vi "Set Endpoints.vi"(8 "Color":u32(colorbox), 9 "B":refnum<class "Point.lvclass">, 10 "A":refnum<class "Point.lvclass">, 11 "Line in":refnum<class "Line example.lvclass">) -> (3 "Line out":refnum<class "Line example.lvclass">)   [LabVIEW 2018, in "Line example.lvclass"]
doc: "Set the endpoints and color of the line."
uses:
  Line example.lvclass
  e:/builds/penguin/labview/branches/2018/dev/dist64/examples/Object-Oriented Programming/Graphics/Graphic/Graphic.lvclass
  Point/Point.lvclass
  Line example.lvclass/Line example.ctl
  Graphic/Graphic.lvclass
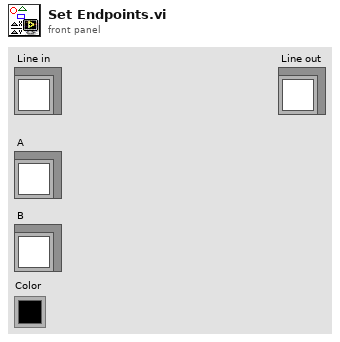
[diagram p1: front panel]
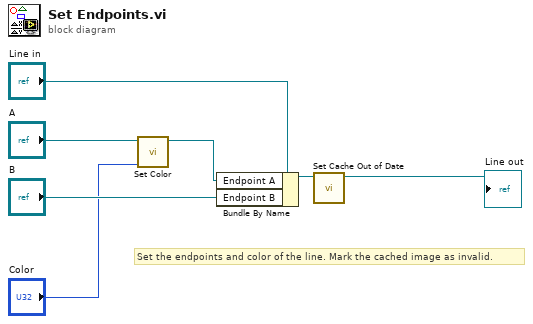
[diagram p0: block diagram]
diagram:
  # "Set the endpoints and color of the line. Mark the cached image as invalid."
  n1 = call "Set Color.vi"("Color"="Color", "Point In"="A") -> ("Point Out"=w1:refnum<class "Point.lvclass">)  [unwired: 9 out]
  n2 = Bundle By Name(cluster="Line in", "Endpoint A"=w1, "Endpoint B"="B") -> (w6:refnum<class "Line example.lvclass">)
  n3 = call "Set Cache Out of Date.vi"("Graphic.lvclass"=w6) -> ("Graphic.lvclass out"=→"Line out":refnum<class "Line example.lvclass">)  [unwired: 10 in]
